vi "Write.vi"(8 "error in (no error)":errorcluster, 9 "Start address":string, 10 "Read Type":variant, 11 "MelsecTCP in":refnum<class "Abs Controler.lvclass">) -> (0 "error out":errorcluster, 3 "MelsecTCP out":refnum<class "Abs Controler.lvclass">)   [LabVIEW 2020, in "HslCommunication.lvlib" / "Abs Controler.lvclass"]
uses:
  Abs Controler.lvclass
  <vilib>/Utility/Data Type/Type Definitions/Data Type.ctl
  E:/Git/Libraries/develop/PLCMonitor/HslCommunication/_Dependenciecs/HslCommunication.dll
  _Dependenciecs/HslCommunication.dll
  <vilib>/Utility/Data Type/NI_Data Type.lvlib
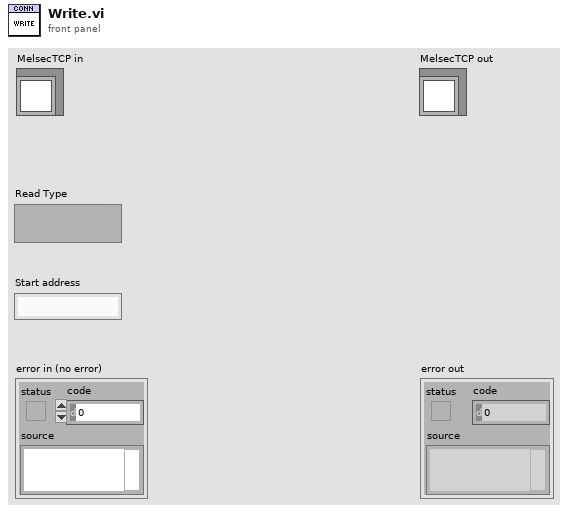
[diagram p1: front panel]
types:
  T1 = typedef "NI_Data Type.lvlib/Data Type.ctl" = enum8{"Invalid Type", "Void", "I8", "I16", "I32", "I64", "U8", "U16", "U32", "U64", "Single Float", "Double Float", "Extended Float", "Single Complex", "Double Complex", "Extended Complex", "Enum U8", "Enum U16", "Enum U32", "Enum U64", "Single Float With Unit", "Double Float With Unit", "Extended Float With Unit", "Single Complex with Unit", "Double Complex with Unit", "Extended Complex with Unit", "Boolean", "String", "Path", "Picture", "Tag", "Array", "Cluster", "Variant", "LV Variant", "Waveform", "Timestamp", "Digital Waveform", "Digital Data", "ExpressData", "Refnum", "External Data", "VI", "Poly VI", "LabVIEW Class Instance", "Fixed Point", "Set Collection", "Map Collection"}
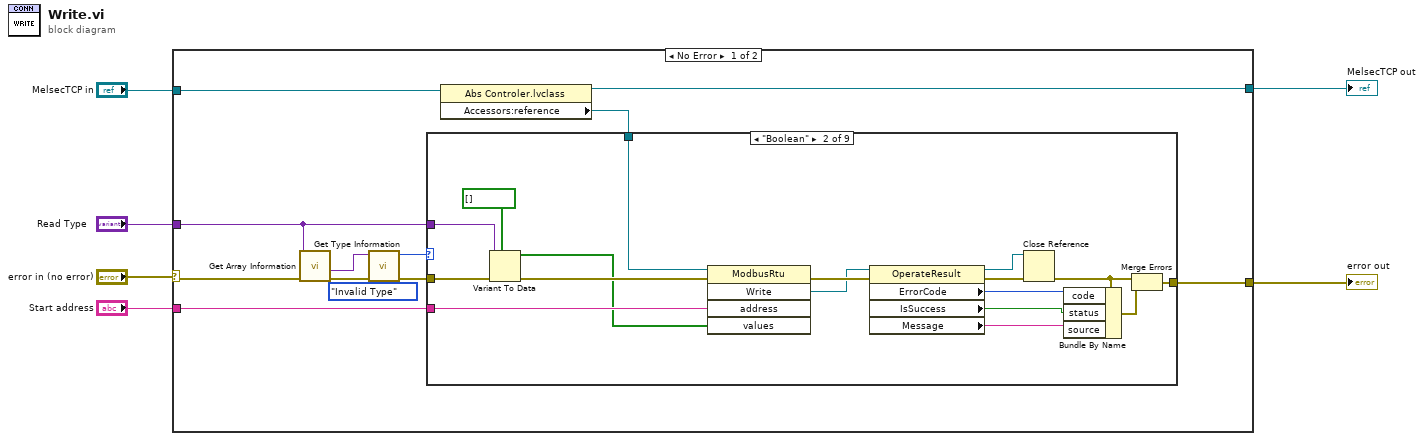
[diagram p0: block diagram]
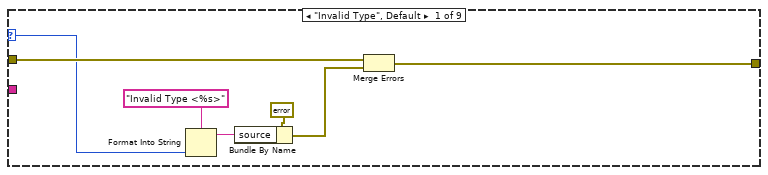
[diagram p2: hidden frame]
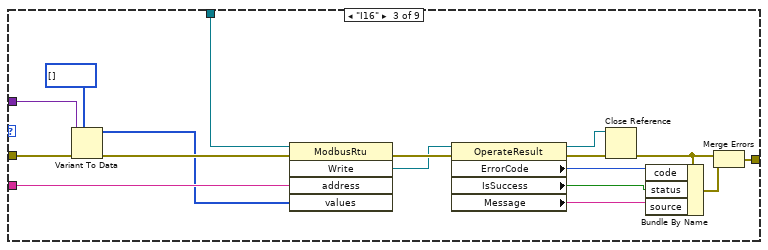
[diagram p3: hidden frame]
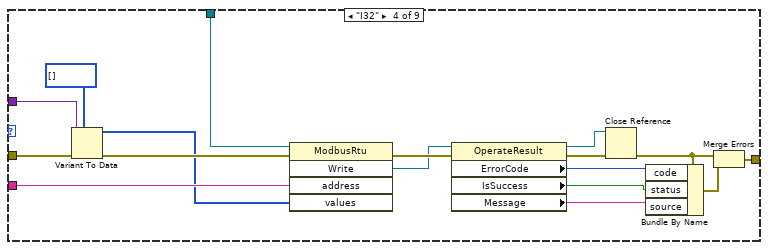
[diagram p4: hidden frame]
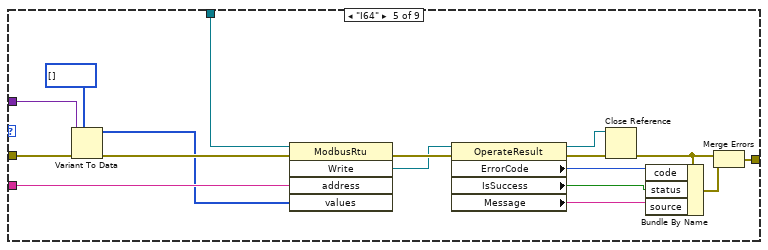
[diagram p5: hidden frame]
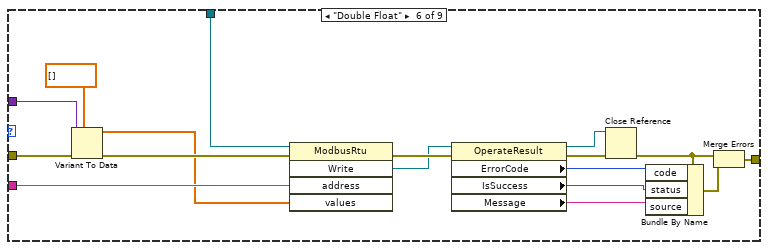
[diagram p6: hidden frame]
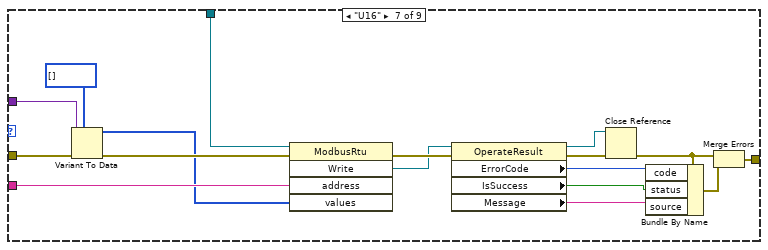
[diagram p7: hidden frame]
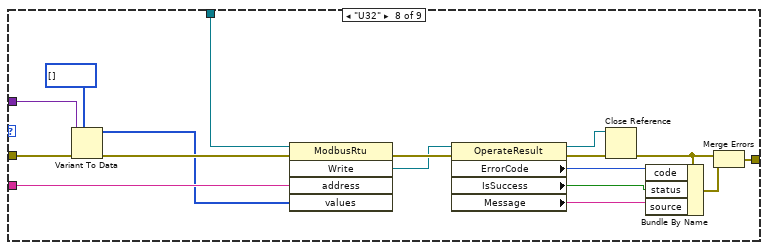
[diagram p8: hidden frame]
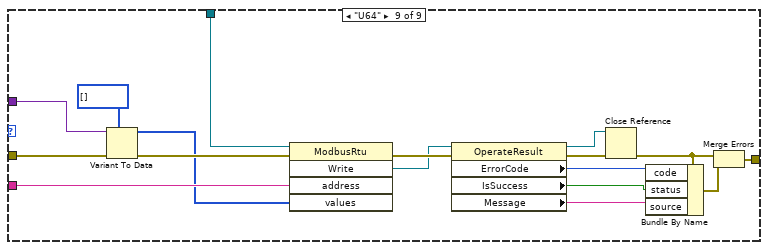
[diagram p9: hidden frame]
diagram:
  n1 = case shown="No Error" "error in (no error)" {
    selector: "error in (no error)" -> [w10 w162]
    tunnel: "MelsecTCP in" -> [w11 w161]
    tunnel: [w16 w161] -> w1
    tunnel: "Start address" -> [w9 _]
    tunnel: [w7 w162] -> w3
    tunnel: "Read Type" -> [w8 _]
    frame No Error {
      (unwired) Data_Type."Invalid Type" ("type")
      n2 = call <vilib>:"Get Array Information.vi"("error in (no error)"=w10, "variant"=w8) -> ("error out"=w14:errorcluster, "array element data type"=w15:variant)  [unwired: 6 in, 2 out]
      n3 = call <vilib>:"Get Type Information.vi"("error in (no error)"=w14, "variant"=w15) -> ("error out"=w13:errorcluster, "type"=w12:T1)  [unwired: 5 in, 3 out]
      n4 = property class="Abs Controler.lvclass"(reference=w11) -> (reference out=w16:refnum<class "Abs Controler.lvclass">, "Accessors:reference"=w17:refnum<k24>)  [unwired: 1 in, 1 out]
      n5 = case shown="\"Boolean\"" w12 {
        selector: w12 -> [w22 _ _ _ _ _ _ _ _]
        tunnel: w17 -> [_ w41 w58 w75 w92 w109 w126 w143 w160]
        tunnel: w9 -> [_ w40 w57 w74 w91 w108 w125 w142 w159]
        tunnel: [w23 w39 w56 w73 w90 w107 w124 w141 w158] -> w7
        tunnel: w8 -> [_ w33 w50 w67 w84 w101 w118 w135 w152]
        tunnel: w13 -> [w24 w32 w49 w66 w83 w100 w117 w134 w151]
        frame "Invalid Type", Default {
          n6 = Format Into String(format string="Invalid Type <%s>", w22) -> (resulting string=w19:string)  [unwired: 2 in, 1 out]
          n7 = Bundle By Name(cluster=errorcluster {"status"=TRUE, "code"=-1, "source"=""} ("error IO"), "source"=w19) -> (w18:errorcluster)
          n8 = Merge Errors(w24, w18) -> (w23:errorcluster)
        }
        frame "Boolean" {
          n9 = Variant To Data(error in=w32, type=bool[] [], Variant=w33) -> (data=w25:bool[], error out=w27:errorcluster)
          n10 = invoke class="ModbusRtu" method="Write"(reference=w41, error in=w27, "address"=w40, "values"=w25) -> (error out=w31:errorcluster, "Write"=w29:refnum<k24>)  [unwired: 1 in, 3 out]
          n11 = property class="OperateResult"(reference=w29, error in=w31) -> (reference out=w28:refnum<k24>, error out=w30:errorcluster, "ErrorCode"=w38:i32, "IsSuccess"=w37:bool, "Message"=w36:string)
          n12 = Close Reference(reference=w28, error in (no error)=w30) -> (error out=w35:errorcluster)
          n13 = Bundle By Name(cluster=w35, "code"=w38, "status"=w37, "source"=w36) -> (w34:errorcluster)
          n14 = Merge Errors(w35, w34) -> (w39:errorcluster)
        }
        frame "I16" {
          n15 = Variant To Data(error in=w49, type=i16[] [], Variant=w50) -> (data=w42:i16[], error out=w44:errorcluster)
          n16 = invoke class="ModbusRtu" method="Write"(reference=w58, error in=w44, "address"=w57, "values"=w42) -> (error out=w48:errorcluster, "Write"=w46:refnum<k24>)  [unwired: 1 in, 3 out]
          n17 = property class="OperateResult"(reference=w46, error in=w48) -> (reference out=w45:refnum<k24>, error out=w47:errorcluster, "ErrorCode"=w55:i32, "IsSuccess"=w54:bool, "Message"=w53:string)
          n18 = Close Reference(reference=w45, error in (no error)=w47) -> (error out=w52:errorcluster)
          n19 = Bundle By Name(cluster=w52, "code"=w55, "status"=w54, "source"=w53) -> (w51:errorcluster)
          n20 = Merge Errors(w52, w51) -> (w56:errorcluster)
        }
        frame "I32" {
          n21 = Variant To Data(error in=w66, type=i32[] [], Variant=w67) -> (data=w59:i32[], error out=w61:errorcluster)
          n22 = invoke class="ModbusRtu" method="Write"(reference=w75, error in=w61, "address"=w74, "values"=w59) -> (error out=w65:errorcluster, "Write"=w63:refnum<k24>)  [unwired: 1 in, 3 out]
          n23 = property class="OperateResult"(reference=w63, error in=w65) -> (reference out=w62:refnum<k24>, error out=w64:errorcluster, "ErrorCode"=w72:i32, "IsSuccess"=w71:bool, "Message"=w70:string)
          n24 = Close Reference(reference=w62, error in (no error)=w64) -> (error out=w69:errorcluster)
          n25 = Bundle By Name(cluster=w69, "code"=w72, "status"=w71, "source"=w70) -> (w68:errorcluster)
          n26 = Merge Errors(w69, w68) -> (w73:errorcluster)
        }
        frame "I64" {
          n27 = Variant To Data(error in=w83, type=i64[] [], Variant=w84) -> (data=w76:i64[], error out=w78:errorcluster)
          n28 = invoke class="ModbusRtu" method="Write"(reference=w92, error in=w78, "address"=w91, "values"=w76) -> (error out=w82:errorcluster, "Write"=w80:refnum<k24>)  [unwired: 1 in, 3 out]
          n29 = property class="OperateResult"(reference=w80, error in=w82) -> (reference out=w79:refnum<k24>, error out=w81:errorcluster, "ErrorCode"=w89:i32, "IsSuccess"=w88:bool, "Message"=w87:string)
          n30 = Close Reference(reference=w79, error in (no error)=w81) -> (error out=w86:errorcluster)
          n31 = Bundle By Name(cluster=w86, "code"=w89, "status"=w88, "source"=w87) -> (w85:errorcluster)
          n32 = Merge Errors(w86, w85) -> (w90:errorcluster)
        }
        frame "Double Float" {
          n33 = Variant To Data(error in=w100, type=dbl[] [], Variant=w101) -> (data=w93:dbl[], error out=w95:errorcluster)
          n34 = invoke class="ModbusRtu" method="Write"(reference=w109, error in=w95, "address"=w108, "values"=w93) -> (error out=w99:errorcluster, "Write"=w97:refnum<k24>)  [unwired: 1 in, 3 out]
          n35 = property class="OperateResult"(reference=w97, error in=w99) -> (reference out=w96:refnum<k24>, error out=w98:errorcluster, "ErrorCode"=w106:i32, "IsSuccess"=w105:bool, "Message"=w104:string)
          n36 = Close Reference(reference=w96, error in (no error)=w98) -> (error out=w103:errorcluster)
          n37 = Bundle By Name(cluster=w103, "code"=w106, "status"=w105, "source"=w104) -> (w102:errorcluster)
          n38 = Merge Errors(w103, w102) -> (w107:errorcluster)
        }
        frame "U16" {
          n39 = Variant To Data(error in=w117, type=u16[] [], Variant=w118) -> (data=w110:u16[], error out=w112:errorcluster)
          n40 = invoke class="ModbusRtu" method="Write"(reference=w126, error in=w112, "address"=w125, "values"=w110) -> (error out=w116:errorcluster, "Write"=w114:refnum<k24>)  [unwired: 1 in, 3 out]
          n41 = property class="OperateResult"(reference=w114, error in=w116) -> (reference out=w113:refnum<k24>, error out=w115:errorcluster, "ErrorCode"=w123:i32, "IsSuccess"=w122:bool, "Message"=w121:string)
          n42 = Close Reference(reference=w113, error in (no error)=w115) -> (error out=w120:errorcluster)
          n43 = Bundle By Name(cluster=w120, "code"=w123, "status"=w122, "source"=w121) -> (w119:errorcluster)
          n44 = Merge Errors(w120, w119) -> (w124:errorcluster)
        }
        frame "U32" {
          n45 = Variant To Data(error in=w134, type=u32[] [], Variant=w135) -> (data=w127:u32[], error out=w129:errorcluster)
          n46 = invoke class="ModbusRtu" method="Write"(reference=w143, error in=w129, "address"=w142, "values"=w127) -> (error out=w133:errorcluster, "Write"=w131:refnum<k24>)  [unwired: 1 in, 3 out]
          n47 = property class="OperateResult"(reference=w131, error in=w133) -> (reference out=w130:refnum<k24>, error out=w132:errorcluster, "ErrorCode"=w140:i32, "IsSuccess"=w139:bool, "Message"=w138:string)
          n48 = Close Reference(reference=w130, error in (no error)=w132) -> (error out=w137:errorcluster)
          n49 = Bundle By Name(cluster=w137, "code"=w140, "status"=w139, "source"=w138) -> (w136:errorcluster)
          n50 = Merge Errors(w137, w136) -> (w141:errorcluster)
        }
        frame "U64" {
          n51 = Variant To Data(error in=w151, type=u64[] [], Variant=w152) -> (data=w144:u64[], error out=w146:errorcluster)
          n52 = invoke class="ModbusRtu" method="Write"(reference=w160, error in=w146, "address"=w159, "values"=w144) -> (error out=w150:errorcluster, "Write"=w148:refnum<k24>)  [unwired: 1 in, 3 out]
          n53 = property class="OperateResult"(reference=w148, error in=w150) -> (reference out=w147:refnum<k24>, error out=w149:errorcluster, "ErrorCode"=w157:i32, "IsSuccess"=w156:bool, "Message"=w155:string)
          n54 = Close Reference(reference=w147, error in (no error)=w149) -> (error out=w154:errorcluster)
          n55 = Bundle By Name(cluster=w154, "code"=w157, "status"=w156, "source"=w155) -> (w153:errorcluster)
          n56 = Merge Errors(w154, w153) -> (w158:errorcluster)
        }
      }
    }
    frame Error {
    }
  }
  "error out" <- w3
  "MelsecTCP out" <- w1
